vi "Project310G05BWeds.vi"() -> ()   [LabVIEW 2016]
uses:
  <vilib>/Utility/file.llb/Read Delimited Spreadsheet (I64).vi
  <vilib>/Utility/file.llb/Write Delimited Spreadsheet (I64).vi
panel:
  in  "File for Counter":path=path "U:/mse 310 project Nov 23/New proj nov 23/CounterArray"
  out "Counter":i64[](array[numeric])
  in  "File for Status":path=path "U:/mse 310 project Nov 23/New proj nov 23/CounterArray"
  out "Status":i64[](array[numeric])
  out "Iteration":i32
  out "Assembly Detect":bool
  in  "EXIT":bool
  out "Bottom Object Sensor End":bool
  out "Bottom Solenoid Sensor":bool
  out "Conveyor end Sensor":bool
  out "Capacitive Sensor":bool
  out "Status":i32[](array[numeric])
  out "Counter":i32[](array[numeric])
  in  "Top belt":bool
  in  "Top Solenoid":bool
  in  "Rotary Solenoid":bool
  in  "Bottom Solenoid":bool
  in  "Conveyor Belt":bool
  out "Bottom Metal Sensor":bool
  out "Bottom Object Sensor Beg":bool
  out "Solenoid Top Sensor":bool
  out "Top Metal Sensor":bool
  out "Top Object Sensor":bool
  out "Stop Button":bool
  out "Start Button":bool
  # "Sensors"
  # "System Data"
  # "Top obj"
  # "Widgets"
  # "Efficiency"
  # "Start"
  # "Stop"
  # "Queue"
  # "Rejects"
  # "Top obj"
  # "Metal"
  # "Hopper"
  # "Capacitive"
  # "Assembly"
  # "Detect"
  # "Reject"
  # "Control"
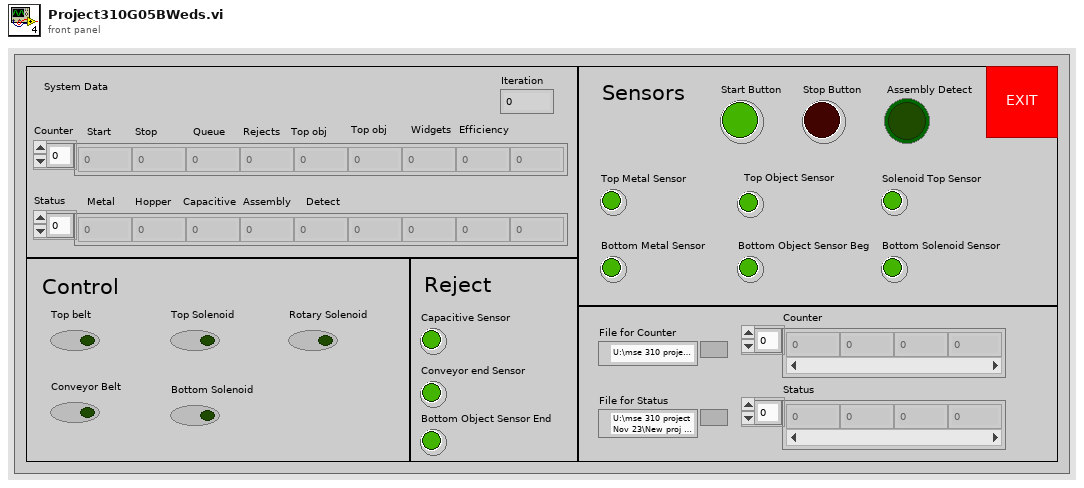
[diagram p1: front panel]
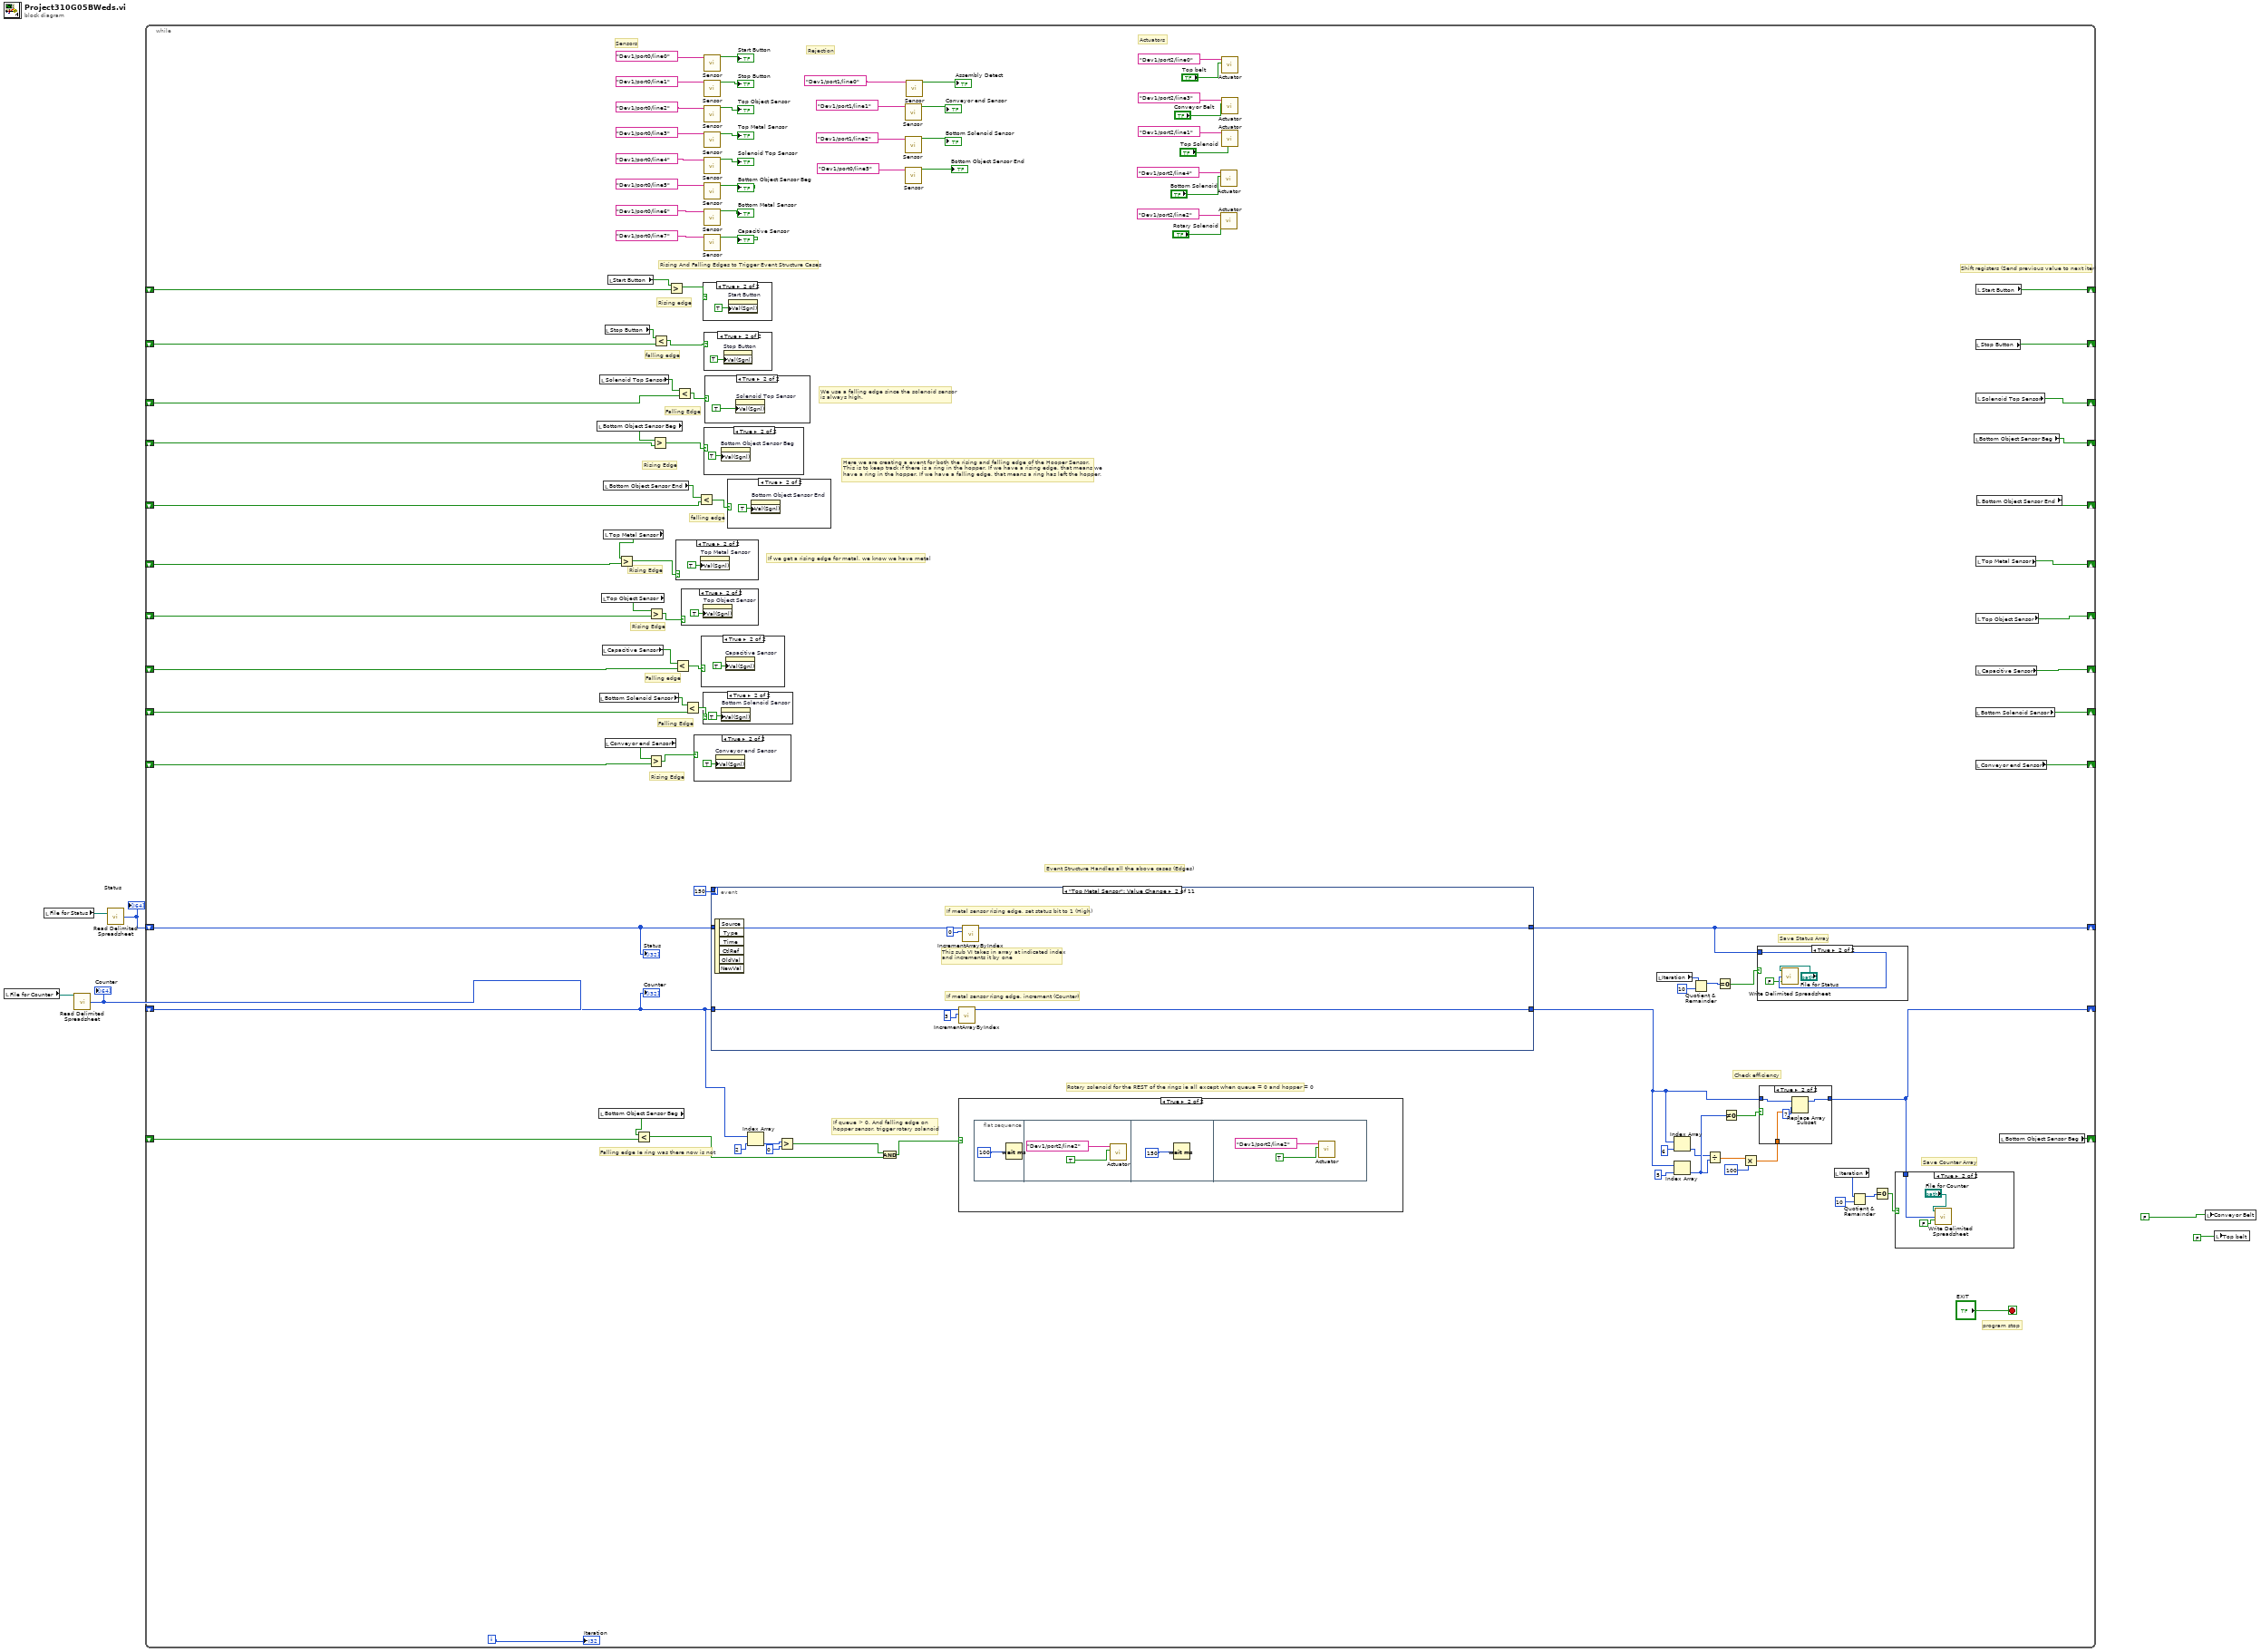
[diagram p0: block diagram]
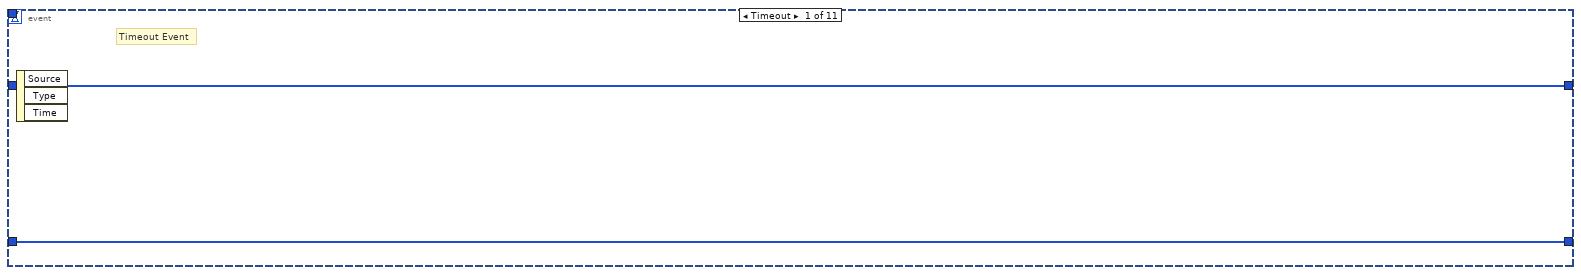
[diagram p16: hidden frame]
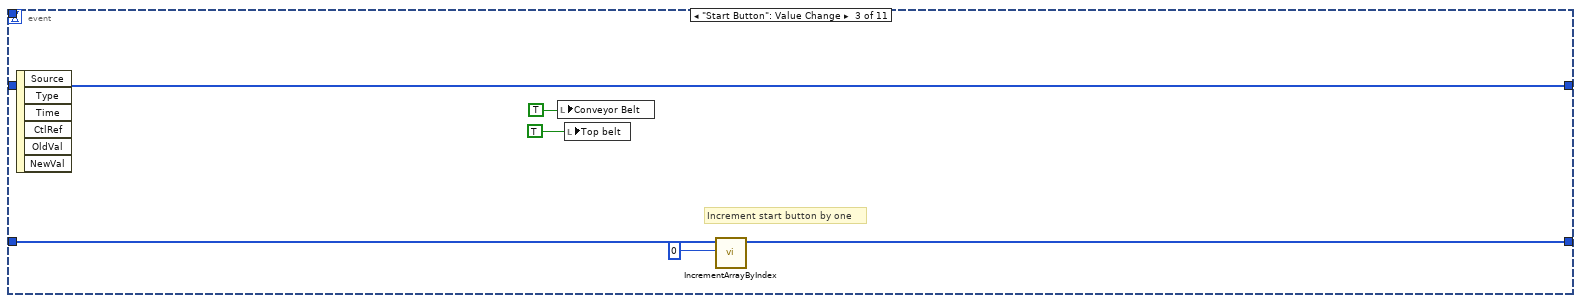
[diagram p17: hidden frame]
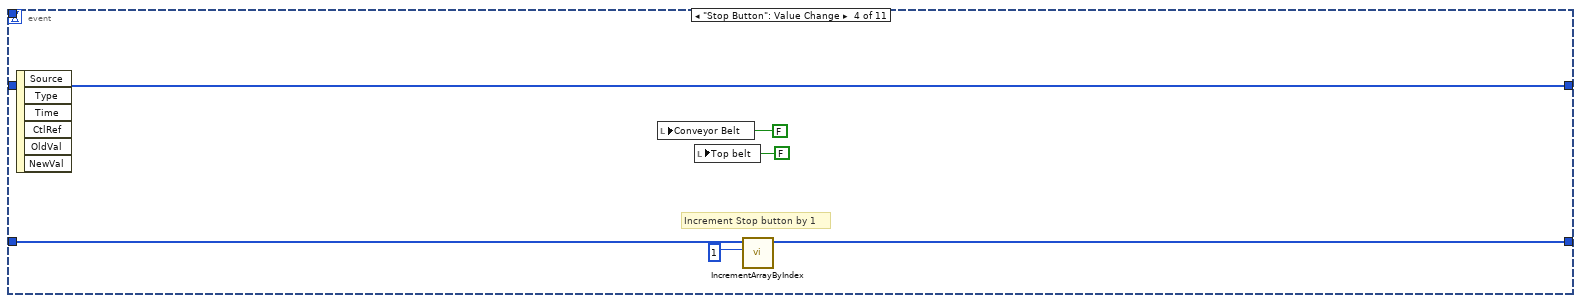
[diagram p18: hidden frame]
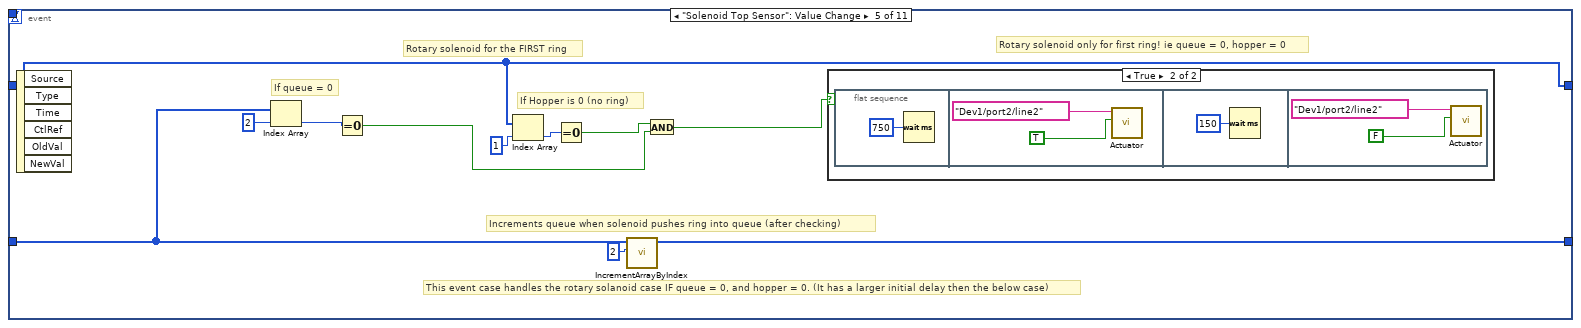
[diagram p19: hidden frame]
diagram:
  n1 = local read "File for Counter"() -> (w2:path)
  n2 = local read "File for Status"() -> (w4:path)
  n3 = call-poly <vilib>:"Read Delimited Spreadsheet.vi"("file path (dialog if empty)"=w2) -> ("first row"=w1:i64[])  [unwired: 9 in, 5 out]
  "Counter" <- w1
  n4 = call-poly <vilib>:"Read Delimited Spreadsheet.vi"("file path (dialog if empty)"=w4) -> ("first row"=w3:i64[])  [unwired: 9 in, 5 out]
  "Status" <- w3
  n5 = while {
    shift-right: [w88] -> _
    shift-left: _ -> [w38]
    shift-right: [w12] -> _
    shift-left: w1 -> [w31]
    shift-right: [w87] -> _
    shift-left: _ -> [w36]
    shift-right: [w86] -> _
    shift-left: _ -> [w43]
    shift-right: [w85] -> _
    shift-left: _ -> [w50]
    shift-right: [w79] -> _
    shift-left: _ -> [w78]
    shift-right: [w7] -> _
    shift-left: w3 -> [w72]
    shift-right: [w73] -> _
    shift-left: _ -> [w74]
    shift-right: [w71] -> _
    shift-left: _ -> [w69]
    shift-right: [w65] -> _
    shift-left: _ -> [w64]
    shift-right: [w55] -> _
    shift-left: _ -> [w54]
    shift-right: [w53] -> _
    shift-left: _ -> [w52]
    shift-right: [w46] -> _
    shift-left: _ -> [w45]
    i -> [w26]
    stop <- "EXIT" stop-if-true
    # "Save Status Array"
    # "Save Counter Array"
    # "Check efficiency"
    # "Sensors"
    # "Shift registers (Send previous value to next iter)"
    # "If queue > 0, And falling edge on\nhopper sensor, trigger rotary solanoid"
    # "Event Structure Handles all the above cases (Edges)"
    # "Falling Edge"
    # "Rising Edge"
    # "Falling edge"
    # "Rising Edge"
    # "If we get a rising edge for metal, we know we have metal"
    # "We use a falling edge since the solenoid sensor\nis always high."
    # "Rising Edge"
    # "Here we are creating a event for both the rising and falling edge of the Hooper Sensor.\nThis is to keep track if there is a ring in the hopper. If we have a rising edge, that means we \nhave a ring in the hopper. If we have a falling edge, that means a ring has left the hopper."
    # "Rising And Falling Edges to Trigger Event Structure Cases"
    # "program stop"
    # "falling edge"
    # "Falling edge Ie ring was there now is not"
    # "Actuators"
    # "Rejection"
    # "Rotary solenoid for the REST of the rings ie all except when queue = 0 and hopper = 0"
    # "Rising Edge"
    # "falling edge"
    # "Falling Edge"
    # "Rising edge"
    n6 = local read "Bottom Object Sensor Beg"() -> (w51:bool)
    n7 = local read "Bottom Object Sensor Beg"() -> (w70:bool)
    n8 = local read "Bottom Solenoid Sensor"() -> (w32:bool)
    n9 = local read "Solenoid Top Sensor"() -> (w37:bool)
    n10 = local read "Top Object Sensor"() -> (w76:bool)
    n11 = local read "Capacitive Sensor"() -> (w33:bool)
    n12 = local read "Bottom Object Sensor End"() -> (w47:bool)
    n13 = local read "Top Metal Sensor"() -> (w77:bool)
    n14 = local read "Stop Button"() -> (w42:bool)
    n15 = local read "Conveyor end Sensor"() -> (w58:bool)
    n16 = local read "Start Button"() -> (w40:bool)
    n17 = Greater?(x=w77, y=w78) -> (0:w34:bool)
    n18 = Less?(x=w70, y=w69) -> (x < y?=w68:bool)
    n19 = Greater?(x=w58, y=w52) -> (0:w57:bool)
    n20 = Greater?(x=w76, y=w74) -> (0:w75:bool)
    n21 = Greater?(x=w51, y=w50) -> (0:w84:bool)
    n22 = Less?(x=w42, y=w43) -> (x < y?=w41:bool)
    n23 = Greater?(x=w40, y=w38) -> (0:w39:bool)
    n24 = Less?(x=w33, y=w64) -> (x < y?=w63:bool)
    n25 = case shown="True" w34 {
      frame False {
      }
      frame True {
        n26 = property on="Top Metal Sensor" class="Bool (strict)"("Val(Sgnl)"=TRUE ("Value (Signaling)")) -> ()  [unwired: 2 in, 2 out]
      }
    }
    n27 = Less?(x=w37, y=w36) -> (x < y?=w35:bool)
    n28 = case shown="True" w75 {
      frame False {
      }
      frame True {
        n29 = property on="Top Object Sensor" class="Bool (strict)"("Val(Sgnl)"=TRUE ("Value (Signaling)")) -> ()  [unwired: 2 in, 2 out]
      }
    }
    n30 = Less?(x=w32, y=w54) -> (x < y?=w56:bool)
    n31 = case shown="True" w57 {
      frame False {
      }
      frame True {
        n32 = property on="Conveyor end Sensor" class="Bool (strict)"("Val(Sgnl)"=TRUE ("Value (Signaling)")) -> ()  [unwired: 2 in, 2 out]
      }
    }
    n33 = Less?(x=w47, y=w45) -> (x < y?=w44:bool)
    n34 = case shown="True" w63 {
      frame False {
      }
      frame True {
        n35 = property on="Capacitive Sensor" class="Bool (strict)"("Val(Sgnl)"=TRUE ("Value (Signaling)")) -> ()  [unwired: 2 in, 2 out]
      }
    }
    n36 = case shown="True" w39 {
      frame False {
      }
      frame True {
        n37 = property on="Start Button" class="Bool (strict)"("Val(Sgnl)"=TRUE ("Value (Signaling)")) -> ()  [unwired: 2 in, 2 out]
      }
    }
    n38 = case shown="True" w56 {
      frame False {
      }
      frame True {
        n39 = property on="Bottom Solenoid Sensor" class="Bool (strict)"("Val(Sgnl)"=TRUE ("Value (Signaling)")) -> ()  [unwired: 2 in, 2 out]
      }
    }
    n40 = case shown="True" w84 {
      frame False {
      }
      frame True {
        n41 = property on="Bottom Object Sensor Beg" class="Bool (strict)"("Val(Sgnl)"=TRUE ("Value (Signaling)")) -> ()  [unwired: 2 in, 2 out]
      }
    }
    n42 = call "Sensor.vi"("lines"=tag "Dev1/port0/line0") -> ("data"=→"Start Button":bool)  [unwired: 10 in]
    n43 = call "Sensor.vi"("lines"=tag "Dev1/port0/line1") -> ("data"=→"Stop Button":bool)  [unwired: 10 in]
    n44 = call "Sensor.vi"("lines"=tag "Dev1/port0/line2") -> ("data"=→"Top Object Sensor":bool)  [unwired: 10 in]
    n45 = call "Sensor.vi"("lines"=tag "Dev1/port0/line3") -> ("data"=→"Top Metal Sensor":bool)  [unwired: 10 in]
    n46 = call "Sensor.vi"("lines"=tag "Dev1/port0/line4") -> ("data"=→"Solenoid Top Sensor":bool)  [unwired: 10 in]
    n47 = call "Sensor.vi"("lines"=tag "Dev1/port0/line5") -> ("data"=→"Bottom Object Sensor Beg":bool)  [unwired: 10 in]
    n48 = call "Sensor.vi"("lines"=tag "Dev1/port0/line6") -> ("data"=→"Bottom Metal Sensor":bool)  [unwired: 10 in]
    n49 = call "Sensor.vi"("lines"=tag "Dev1/port0/line7") -> ("data"=→"Capacitive Sensor":bool)  [unwired: 10 in]
    n50 = case shown="True" w41 {
      frame False {
      }
      frame True {
        n51 = property on="Stop Button" class="Bool (strict)"("Val(Sgnl)"=TRUE ("Value (Signaling)")) -> ()  [unwired: 2 in, 2 out]
      }
    }
    n52 = case shown="True" w35 {
      frame False {
      }
      frame True {
        n53 = property on="Solenoid Top Sensor" class="Bool (strict)"("Val(Sgnl)"=TRUE) -> ()  [unwired: 2 in, 2 out]
      }
    }
    n54 = event shown="[1] \"Top Metal Sensor\": Value Change" {
      selector: _ -> [_ _ _ _ _ _ _ _ _ _ _]
      dyn-events: _ -> [_ _ _ _ _ _ _ _ _ _ _]
      timeout: 150 -> [w142 _ _ _ _ _ _ _ _ _ _]
      tunnel: w31 -> [w143 w149 w154 w159 w169 w179 w188 w201 w208 w218 w229]
      tunnel: [w143 w148 w153 w158 w171 w179 w188 w200 w206 w223 w229] -> w13
      tunnel: [w142 _ _ _ _ _ _ _ _ _ _] -> _
      tunnel: w72 -> [w141 w146 w150 w156 w168 w182 w184 w202 w205 w212 w233]
      tunnel: [w141 w144 w150 w156 w168 w181 w183 w202 w204 w211 w232] -> w7
      event Timeout {
        # "Timeout Event"
        n55 = event-data() -> ()  [unwired: 1 in, 3 out]
      }
      event "Top Metal Sensor": Value Change {
        # "This sub VI takes in array at indicated index\nand increments it by one"
        # "If metal sensor risng edge, increment (Counter)"
        # "If metal sensor rising edge, set status bit to 1 (High)"
        n56 = event-data() -> ()  [unwired: 1 in, 6 out]
        n57 = call "IncrementArrayByIndex.vi"("index"=3, "Array in"=w149) -> ("Array out"=w148:i32[])  [unwired: 9 in]
        n58 = call "IncrementArrayByIndex.vi"("index"=0, "Array in"=w146) -> ("Array out"=w144:i32[])  [unwired: 9 in]
      }
      event "Start Button": Value Change {
        # "Increment start button by one"
        n59 = event-data() -> ()  [unwired: 1 in, 6 out]
        n60 = local write "Conveyor Belt"(TRUE ("Conveyor Belt")) -> ()
        n61 = local write "Top belt"(TRUE) -> ()
        n62 = call "IncrementArrayByIndex.vi"("index"=0, "Array in"=w154) -> ("Array out"=w153:i32[])  [unwired: 9 in]
      }
      event "Stop Button": Value Change {
        # "Increment Stop button by 1"
        n63 = event-data() -> ()  [unwired: 1 in, 6 out]
        n64 = local write "Conveyor Belt"(FALSE ("Conveyor Belt")) -> ()
        n65 = local write "Top belt"(FALSE) -> ()
        n66 = call "IncrementArrayByIndex.vi"("index"=1, "Array in"=w159) -> ("Array out"=w158:i32[])  [unwired: 9 in]
      }
      event "Solenoid Top Sensor": Value Change {
        # "If Hopper is 0 (no ring)"
        # "If queue = 0"
        # "This event case handles the rotary solanoid case IF queue = 0, and hopper = 0. (It has a larger initial delay then the below case)"
        # "Rotary solenoid only for first ring! ie queue = 0, hopper = 0"
        # "Rotary solenoid for the FIRST ring"
        # "Increments queue when solenoid pushes ring into queue (after checking)"
        n67 = event-data() -> ()  [unwired: 1 in, 6 out]
        n68 = Index Array(array=w169, index=2) -> (element=w164:i64)
        n69 = Equal To 0?(x=w164) -> (x = 0?=w162:bool)
        n70 = Index Array(array=w168, index=1) -> (element=w165:i64)
        n71 = Equal To 0?(x=w165) -> (x = 0?=w163:bool)
        n72 = call "IncrementArrayByIndex.vi"("index"=2, "Array in"=w169) -> ("Array out"=w171:i32[])  [unwired: 9 in]
        n73 = And(x=w163, y=w162) -> (x .and. y?=w166:bool)
        n74 = case shown="True" w166 {
          frame False {
          }
          frame True {
            n75 = flat-sequence {
              frame #0 {
                n76 = Wait (ms)(milliseconds to wait=u32 750) -> ()  [unwired: 1 out]
              }
              frame #1 {
                n77 = call "Actuator.vi"("Actuator"=TRUE, "lines"=tag "Dev1/port2/line2") -> ()  [unwired: 10 in]
              }
              frame #2 {
                n78 = Wait (ms)(milliseconds to wait=u32 150) -> ()  [unwired: 1 out]
              }
              frame #3 {
                n79 = call "Actuator.vi"("Actuator"=FALSE, "lines"=tag "Dev1/port2/line2") -> ()  [unwired: 10 in]
              }
            }
          }
        }
      }
      event "Capacitive Sensor": Value Change {
        # "Set capacitive high"
        n80 = event-data() -> ()  [unwired: 1 in, 6 out]
        n81 = call "IncrementArrayByIndex.vi"("index"=2, "Array in"=w182) -> ("Array out"=w181:i32[])  [unwired: 9 in]
      }
      event "Conveyor end Sensor": Value Change {
        # "If capacitive sensor bit = low"
        # "In this Event case we activate the lower solenoid IF capacitive sensor is low, sets capacitive to zero if false"
        n82 = event-data() -> ()  [unwired: 1 in, 6 out]
        n83 = Index Array(array=w184, index=2) -> (element=w186:i64)
        n84 = Equal To 0?(x=w186) -> (x = 0?=w185:bool)
        n85 = case shown="False" w185 {
          tunnel: w184 -> [w192 w193]
          tunnel: [w189 w193] -> w183
          frame False {
            # "If capacitive sensor is High, dont trigger solenoid and set the capacitive \nbit back to zero."
            n86 = Replace Array Subset(array=w192, new element=0, index=2) -> (w189:i64[])
          }
          frame True {
            # "Activate top solenoid"
            n87 = flat-sequence {
              frame #0 {
                n88 = call "Actuator.vi"("Actuator"=TRUE, "lines"=tag "Dev1/port2/line4") -> ()  [unwired: 10 in]
              }
              frame #1 {
                n89 = Wait (ms)(milliseconds to wait=u32 50) -> ()  [unwired: 1 out]
              }
              frame #2 {
                n90 = call "Actuator.vi"("Actuator"=FALSE, "lines"=tag "Dev1/port2/line4") -> ()  [unwired: 10 in]
              }
            }
          }
        }
      }
      event "Bottom Solenoid Sensor": Value Change {
        # "This means something was rejected,\nthus increment reject counter"
        n91 = event-data() -> ()  [unwired: 1 in, 6 out]
        n92 = call "IncrementArrayByIndex.vi"("index"=3, "Array in"=w201) -> ("Array out"=w200:i32[])  [unwired: 9 in]
      }
      event "Bottom Object Sensor Beg": Value Change {
        # "Set hopper status to full (high)"
        # "This event structure is for the rising edge of the hopper, ie just got a plastic ring"
        # "Decrements queue when hopper pulls ring from queue"
        n93 = event-data() -> ()  [unwired: 1 in, 6 out]
        n94 = call "IncrementArrayByIndex.vi"("index"=1, "Array in"=w205) -> ("Array out"=w204:i32[])  [unwired: 9 in]
        n95 = call "DecrementArrayByIndex.vi"("index"=2, "Array in"=w208) -> ("Array out"=w206:i32[])  [unwired: 9 in]
      }
      event "Top Object Sensor": Value Change {
        # "Counts how many object passed sensor (not used)"
        # "After checking metal status\nset metal status to zero"
        # "If metal status is zero"
        # "If Queue < 5"
        # "This event case triggers the top solenoid (if its a plastic ring AND queue <5)"
        n96 = event-data() -> ()  [unwired: 1 in, 6 out]
        n97 = Index Array(array=w212, index=0) -> (element=w220:i64)
        n98 = Index Array(array=w218, index=2) -> (element=w216:i64)
        n99 = Equal To 0?(x=w220) -> (x = 0?=w217:bool)
        n100 = Less?(x=w216, y=5) -> (x < y?=w214:bool)
        n101 = And(x=w217, y=w214) -> (x .and. y?=w213:bool)
        n102 = Replace Array Subset(array=w212, new element=0, index=0) -> (w211:i64[])
        n103 = call "IncrementArrayByIndex.vi"("index"=4, "Array in"=w218) -> ("Array out"=w223:i32[])  [unwired: 9 in]
        n104 = case shown="True" w213 {
          frame False {
          }
          frame True {
            n105 = flat-sequence {
              frame #0 {
                n106 = call "Actuator.vi"("Actuator"=TRUE, "lines"=tag "Dev1/port2/line1") -> ()  [unwired: 10 in]
              }
              frame #1 {
                n107 = Wait (ms)(milliseconds to wait=u32 50) -> ()  [unwired: 1 out]
              }
              frame #2 {
                n108 = call "Actuator.vi"("Actuator"=FALSE, "lines"=tag "Dev1/port2/line1") -> ()  [unwired: 10 in]
              }
            }
          }
        }
      }
      event "Bottom Object Sensor End": Value Change {
        # "Set hopper status to zero (empty)"
        # "This event case is for the falling edge of the hopper, ie ring just leaves hopper."
        n109 = event-data() -> ()  [unwired: 1 in, 6 out]
        n110 = Replace Array Subset(array=w233, new element=0, index=1) -> (w232:i64[])
      }
    }
    n111 = case shown="True" w44 {
      frame False {
      }
      frame True {
        n112 = property on="Bottom Object Sensor End" class="Bool (strict)"("Val(Sgnl)"=TRUE ("Value (Signaling)")) -> ()  [unwired: 2 in, 2 out]
      }
    }
    n113 = Index Array(array=w31, index=2) -> (element=w81:i64)
    n114 = Greater?(x=w81, y=0) -> (0:w30:bool)
    n115 = And(x=w30, y=w68) -> (x .and. y?=w82:bool)
    n116 = call "Sensor.vi"("lines"=tag "Dev1/port1/line1") -> ("data"=→"Conveyor end Sensor":bool)  [unwired: 10 in]
    n117 = call "Sensor.vi"("lines"=tag "Dev1/port1/line2") -> ("data"=→"Bottom Solenoid Sensor":bool)  [unwired: 10 in]
    n118 = call "Sensor.vi"("lines"=tag "Dev1/port0/line5") -> ("data"=→"Bottom Object Sensor End":bool)  [unwired: 10 in]
    n119 = call "Sensor.vi"("lines"=tag "Dev1/port1/line0") -> ("data"=→"Assembly Detect":bool)  [unwired: 10 in]
    n120 = case shown="True" w82 {
      frame False {
      }
      frame True {
        n121 = flat-sequence {
          frame #0 {
            n122 = Wait (ms)(milliseconds to wait=100) -> ()  [unwired: 1 out]
          }
          frame #1 {
            n123 = call "Actuator.vi"("Actuator"=TRUE, "lines"=tag "Dev1/port2/line2") -> ()  [unwired: 10 in]
          }
          frame #2 {
            n124 = Wait (ms)(milliseconds to wait=150) -> ()  [unwired: 1 out]
          }
          frame #3 {
            n125 = call "Actuator.vi"("Actuator"=TRUE, "lines"=tag "Dev1/port2/line2") -> ()  [unwired: 10 in]
          }
        }
      }
    }
    n126 = call "Actuator.vi"("Actuator"="Bottom Solenoid", "lines"=tag "Dev1/port2/line4") -> ()  [unwired: 10 in]
    n127 = call "Actuator.vi"("Actuator"="Rotary Solenoid", "lines"=tag "Dev1/port2/line2") -> ()  [unwired: 10 in]
    n128 = call "Actuator.vi"("Actuator"="Top belt", "lines"=tag "Dev1/port2/line0") -> ()  [unwired: 10 in]
    n129 = call "Actuator.vi"("Actuator"="Conveyor Belt", "lines"=tag "Dev1/port2/line3") -> ()  [unwired: 10 in]
    n130 = call "Actuator.vi"("Actuator"="Top Solenoid", "lines"=tag "Dev1/port2/line1") -> ()  [unwired: 10 in]
    n131 = local read "Iteration"() -> (w11:i32)
    n132 = Index Array(array=w13, index=6) -> (element=w20:i64)
    n133 = Index Array(array=w13, index=5) -> (element=w21:i64)
    n134 = Quotient & Remainder(x=w11, y=10) -> (x-y*floor(x/y)=w9:i32)  [unwired: 1 out]
    n135 = Divide(x=w20, y=w21) -> (x/y=w23:dbl)
    n136 = Equal To 0?(x=w9) -> (x = 0?=w10:bool)
    n137 = Not Equal To 0?(x=w21) -> (x != 0?=w22:bool)
    n138 = Multiply(x=w23, y=100) -> (x*y=w25:dbl)
    n139 = case shown="True" w10 {
      tunnel: w7 -> [_ w116]
      frame False {
      }
      frame True {
        n140 = call-poly <vilib>:"Write Delimited Spreadsheet.vi"("file path (dialog if empty)"="File for Status", "1D data"=w116, "append to file? (new file:F)"=FALSE) -> ()  [unwired: 11 in, 2 out]
      }
    }
    n141 = case shown="True" w22 {
      tunnel: w13 -> [w120 w122]
      tunnel: [w120 w123] -> w12
      tunnel: w25 -> [_ w121]
      frame False {
      }
      frame True {
        n142 = Replace Array Subset(array=w122, new element=w121, index=7) -> (w123:i64[])
      }
    }
    n143 = local read "Iteration"() -> (w14:i32)
    n144 = Quotient & Remainder(x=w14, y=10) -> (x-y*floor(x/y)=w16:i32)  [unwired: 1 out]
    n145 = Equal To 0?(x=w16) -> (x = 0?=w17:bool)
    n146 = case shown="True" w17 {
      tunnel: w12 -> [_ w119]
      frame False {
      }
      frame True {
        n147 = call-poly <vilib>:"Write Delimited Spreadsheet.vi"("file path (dialog if empty)"="File for Counter", "1D data"=w119, "append to file? (new file:F)"=FALSE) -> ()  [unwired: 11 in, 2 out]
      }
    }
    n148 = local read "Bottom Object Sensor Beg"() -> (w85:bool)
    n149 = local read "Stop Button"() -> (w86:bool)
    n150 = local read "Bottom Solenoid Sensor"() -> (w55:bool)
    n151 = local read "Conveyor end Sensor"() -> (w53:bool)
    n152 = local read "Start Button"() -> (w88:bool)
    n153 = local read "Solenoid Top Sensor"() -> (w87:bool)
    n154 = local read "Top Metal Sensor"() -> (w79:bool)
    n155 = local read "Top Object Sensor"() -> (w73:bool)
    n156 = local read "Capacitive Sensor"() -> (w65:bool)
    n157 = local read "Bottom Object Sensor End"() -> (w46:bool)
    n158 = local read "Bottom Object Sensor Beg"() -> (w71:bool)
    "Counter" <- w31
    "Status" <- w72
    "Iteration" <- w26
  }
  n159 = local write "Conveyor Belt"(FALSE ("Conveyor Belt")) -> ()
  n160 = local write "Top belt"(FALSE ("Top belt")) -> ()
